vi "Set Destination Path.vi"(8 "error in (no error)":errorcluster, 9 "Destination path":path, 10 "Destination label":string, 11 "DLL in":refnum<class "NI_AB_API_DLL.lvclass">) -> (0 "error out":errorcluster, 3 "DLL out":refnum<class "NI_AB_API_DLL.lvclass">)   [LabVIEW 2020, in "NI_AB_API_DLL.lvclass"]
uses:
  <vilib>/AppBuilder/AB_API/DLL/NI_AB_API_DLL.lvclass
  <vilib>/AppBuilder/AB_API/Application/NI_AB_API_Application.lvclass
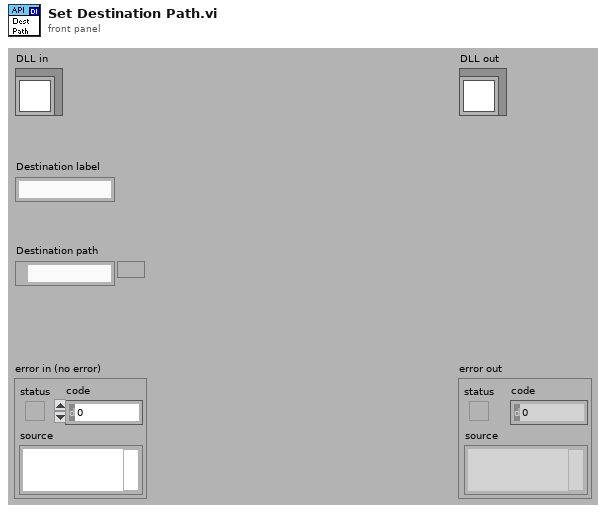
[diagram p1: front panel]
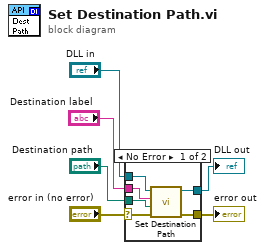
[diagram p0: block diagram]
diagram:
  n1 = case shown="No Error" "error in (no error)" {
    selector: "error in (no error)" -> [w8 w14]
    tunnel: [w7 w14] -> w2
    tunnel: [w11 w13] -> w1
    tunnel: "DLL in" -> [w12 w13]
    tunnel: "Destination label" -> [w9 _]
    tunnel: "Destination path" -> [w10 _]
    frame No Error {
      n2 = call-parent "Set Destination Path.vi"("error in (no error)"=w8, "Destination path"=w10, "Destination label"=w9, "Build in"=w12) -> ("error out"=w7:errorcluster, "Build out"=w11:refnum<class "NI_AB_API_DLL.lvclass">)  [unwired: 6 in]
    }
    frame Error {
    }
  }
  "error out" <- w2
  "DLL out" <- w1
